vi "UpdateTimesStim.vi"(8 "error in (no error)":errorcluster, 11 "Stim in":refnum<class "Stim.lvclass">) -> (0 "error out":errorcluster, 1 "Trial":dbl, 2 "Juice":bool[](array[boolean]), 3 "Stim out":refnum<class "Stim.lvclass">, 4 "Stimulus":string, 5 "New trial":bool)   [LabVIEW 2014, in "Stim.lvclass"]
uses:
  Stim.lvclass
  Stim.lvclass/Stim.ctl
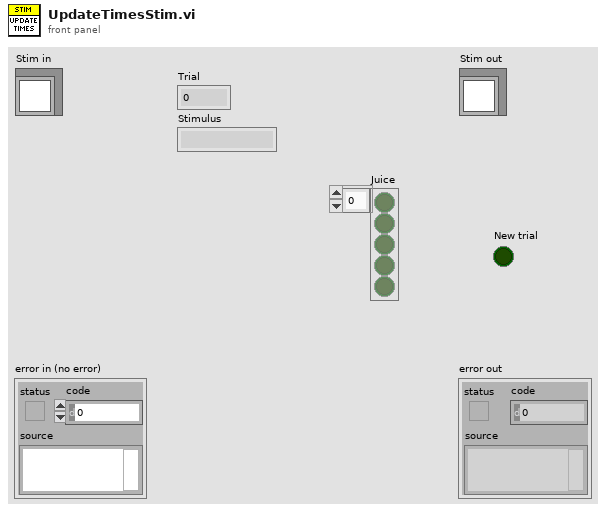
[diagram p1: front panel]
types:
  T1 = cluster{"Stimulus channels":bool[], "Stimulus":string}
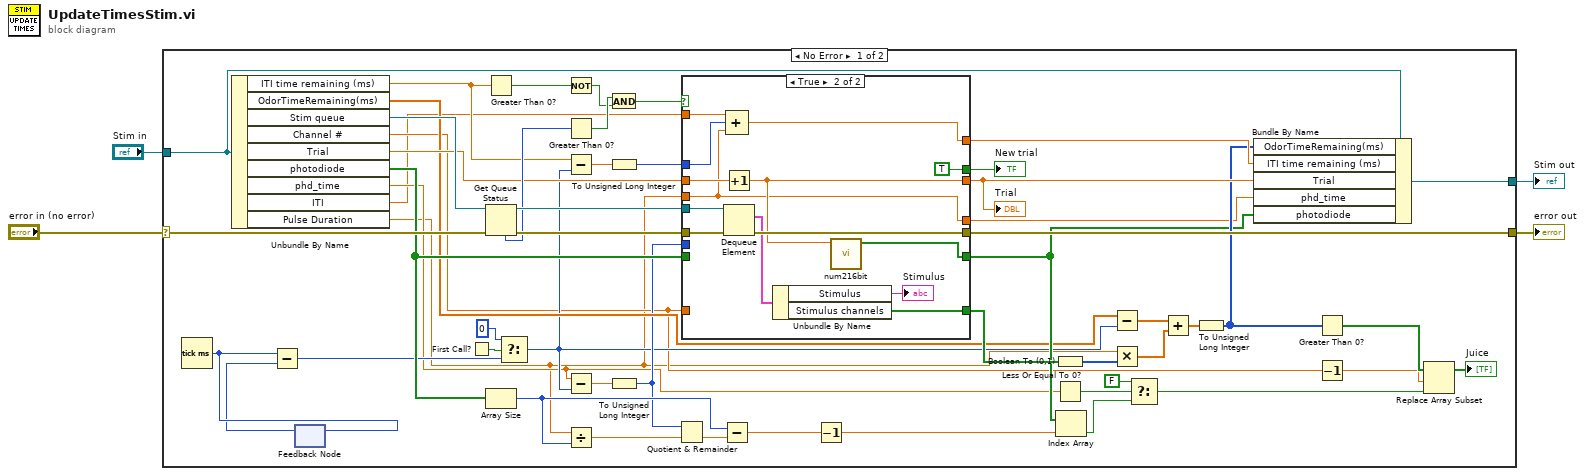
[diagram p0: block diagram]
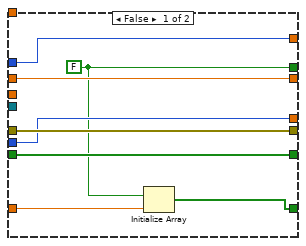
[diagram p2: hidden frame]
diagram:
  n1 = case shown="No Error" "error in (no error)" {
    selector: "error in (no error)" -> [w50 w81]
    tunnel: [w49 w81] -> w2
    tunnel: [w42 w80] -> w1
    tunnel: "Stim in" -> [w43 w80]
    frame No Error {
      n2 = Tick Count (ms)() -> (millisecond timer value=w57:u32)
      n3 = Unbundle By Name(w43) -> ("ITI time remaining (ms)"=w22:dbl, "OdorTimeRemaining(ms)"=w25:dbl[], "Stim queue"=w54:refnum<queue>, "Channel #"=w8:dbl, "Trial"=w38:dbl, "photodiode"=w33:bool[], "phd_time"=w11:dbl, "ITI"=w5:dbl, "Pulse Duration"=w6:dbl)
      n4 = feedback-in #1(w57) -> ()
      n5 = feedback #1() -> (w56:u32)  [unwired: 1 in]
      n6 = Subtract(x=w57, y=w56) -> (x-y=w21:u32)
      n7 = First Call?() -> (First Call?: T/F=w18:bool)
      n8 = Greater Than 0?(x=w22) -> (x > 0?=w15:bool)
      n9 = Get Queue Status(queue=w54, error in (no error)=w50) -> (queue out=w53:refnum<queue>, error out=w52:errorcluster, # elements in queue=w51:i32)  [unwired: 1 in, 5 out]
      n10 = Array Size(array=w33) -> (size(s)=w27:i32)
      n11 = Select(t=u32 0, s=w18, f=w21) -> (s? t:f=w20:u32)
      n12 = Not(x=w15) -> (.not. x?=w44:bool)
      n13 = Greater Than 0?(x=w51) -> (x > 0?=w47:bool)
      n14 = Subtract(x=w22, y=w20) -> (x-y=w45:dbl)
      n15 = Subtract(x=w11, y=w20) -> (x-y=w34:dbl)
      n16 = Divide(x=w6, y=w27) -> (x/y=w26:dbl)
      n17 = And(x=w47, y=w44) -> (x .and. y?=w46:bool)
      n18 = To Unsigned Long Integer(number=w45) -> (unsigned 32bit integer=w37:u32)
      n19 = To Unsigned Long Integer(number=w34) -> (unsigned 32bit integer=w23:u32)
      n20 = Quotient & Remainder(x=w23, y=w26) -> (floor(x/y)=w28:dbl)  [unwired: 1 out]
      n21 = case shown="True" w46 {
        tunnel: [w65 w79] -> w49
        tunnel: w53 -> [_ w78]
        tunnel: w52 -> [w65 w77]
        tunnel: [w63 w75] -> w32
        tunnel: w8 -> [w64 _]
        tunnel: [w62 w71] -> w39
        tunnel: w38 -> [w62 w74]
        tunnel: w37 -> [w61 w73]
        tunnel: w6 -> [_ w69]
        tunnel: [w61 w72] -> w36
        tunnel: w33 -> [w60 _]
        tunnel: [w60 w70] -> w29
        tunnel: [w59 w69] -> w24
        tunnel: w23 -> [w59 _]
        tunnel: [w58 TRUE] -> w7
        tunnel: w5 -> [_ w66]
        frame False {
          w58 = FALSE
          n22 = Initialize Array(w58, w64) -> (w63:bool[])
        }
        frame True {
          n23 = Increment(x=w74) -> (x+1=w71:dbl)
          n24 = Dequeue Element(queue=w78, error in (no error)=w77) -> (element=w76:T1, error out=w79:errorcluster)  [unwired: 1 in, 2 out]
          n25 = Compound Arithmetic op=ADD(w66, w73, w69) -> (w72:dbl)
          n26 = Unbundle By Name(w76) -> ("Stimulus"=→"Stimulus":string, "Stimulus channels"=w75:bool[])
          n27 = call "num216bit.vi"("Trial#"=w71) -> ("phd_array"=w70:bool[])  [unwired: 10 in]
        }
      }
      "Trial" <- w39
      "New trial" <- w7
      n28 = Subtract(x=w27, y=w28) -> (x-y=w17:dbl)
      n29 = Decrement(x=w17) -> (x-1=w16:dbl)
      n30 = Boolean To (0,1)(Boolean=w32) -> (0, 1=w41:i16[])
      n31 = Less Or Equal To 0?(x=w11) -> (x <= 0?=w10:bool)
      n32 = Index Array(array=w29, index=w16) -> (element=w13:bool)
      n33 = Subtract(x=w25, y=w20) -> (x-y=w55:dbl[])
      n34 = Multiply(x=w6, y=w41) -> (x*y=w48:dbl[])
      n35 = Select(t=FALSE, s=w10, f=w13) -> (s? t:f=w12:bool)
      n36 = Add(x=w55, y=w48) -> (x+y=w40:dbl[])
      n37 = To Unsigned Long Integer(number=w40) -> (unsigned 32bit integer=w35:u32[])
      n38 = Bundle By Name(cluster=w43, "OdorTimeRemaining(ms)"=w35, "ITI time remaining (ms)"=w36, "Trial"=w39, "phd_time"=w24, "photodiode"=w29) -> (w42:refnum<class "Stim.lvclass">)
      n39 = Greater Than 0?(x=w35) -> (x > 0?=w31:bool[])
      n40 = Decrement(x=w8) -> (x-1=w9:dbl)
      n41 = Replace Array Subset(array=w31, new element=w12, index=w9) -> (→"Juice":bool[])
    }
    frame Error {
    }
  }
  "error out" <- w2
  "Stim out" <- w1
